vi "远端校准.vi"   [LabVIEW 2016, in "MB SLAVE.lvlib"]
uses:
  MB SLAVE.lvlib
  <vilib>/Plasmionique/MB Master/MB_Master/MB_Master.lvclass
  <vilib>/Plasmionique/MB Master/MB Master.lvlib
types:
  T1 = typedef "MB SLAVE.lvlib/启动命令类型.ctl" = enum16{"启动整机", "停止整机", "标样核查", "加标回收", "平行样测试", "零点核查", "跨度核查", "校零", "校标", "启动系统全面清洗", "水样测试", "启动采水泵阀", "校准", "仪器重启"}
  T2 = cluster{"启动类型":T1, "启动参数":enum16{"未选择", "CODMn", "氨氮", "总磷", "总氮", "CODCr"}}
  T3 = enum16{"未选择", "CODMn", "氨氮", "总磷", "总氮", "CODCr"}
  T4 = typedef "CODMn交互.ctl" = cluster{"COD浓度（mg/L)":dbl, "水样启动时间":timestamp, "加标回收启动时间":timestamp, "CODMn工作状态":enum16{"空闲", "水样测试", "标样核查", "零点核查", "跨度核查", "空白测试", "平行样测试", "加标回收", "空白校准", "标样校准", "初始化（清洗）"}, "多列列表框":i32, "平台试剂余量百分比":sgl, "关键参数":cluster{"测量量程":dbl, "测量精度":dbl, "测量间隔":dbl, "消解温度":dbl, "消解时长":dbl, "空白校准时间":timestamp, "曲线截距":dbl, "曲线斜率":dbl, "测量检出限":dbl, "测量信号值":dbl, "线性相关系数":dbl, "二次多项式系数":dbl, "标样校准时间":timestamp, "稀释倍数":dbl, "三项式系数":dbl, "空白标定系数":dbl, "量程系数":dbl, "F0/ORPA":dbl, "F1/ORPB":dbl, "F2/ORPK":dbl, "F3":dbl, "F4":dbl, "F5":dbl, "F6":dbl, "F7":dbl, "X0/滴定数":dbl, "量程":dbl}, "关键参数改变":bool, "校准信息":cluster{"低标液1浓度":dbl, "低标液1信号值":dbl, "低标液1启用":u16, "低标液2浓度":dbl, "低标液2信号值":dbl, "低标液2启用":u16, "低标液3浓度":dbl, "低标液3信号值":dbl, "低标液3启用":u16, "低标液4浓度":dbl, "低标液4信号值":dbl, "低标液4启用":u16, "低标液5浓度":dbl, "低标液5信号值":dbl, "低标液5启用":u16, "高标液1浓度":dbl, "高标液1信号值":dbl, "高标液1启用":u16, "高标液2浓度":dbl, "高标液2信号值":dbl, "高标液2启用":u16, "高标液3浓度":dbl, "高标液3信号值":dbl, "高标液3启用":u16, "高标液4浓度":dbl, "高标液4信号值":dbl, "高标液4启用":u16, "高标液5浓度":dbl, "高标液5信号值":dbl, "高标液5启用":u16, "低斜率":dbl, "低截距":dbl, "低二次多项式系数":dbl, "低线性相关系数":dbl, "高斜率":dbl, "高截距":dbl, "高二次多项式系数":dbl, "高线性相关系数":dbl}, "校准信息改变":bool, "固件版本号":string, "CODMn模块版本":T5, "协议":u16, "状态告警区":cluster{"系统时间":timestamp, "工作状态":u16, "测量模式":enum16{"待机", "连续模式", "周期模式", "定点模式", "受控模式", "手动模式"}, "告警代码":u16, "故障代码":u16, "日志代码":u16, "软件版本":u16, "F0":sgl, "F1":sgl, "F2":sgl, "F3":sgl, "T":sgl, "H":sgl, "id":u16, "flowid":u16, "量程":u16, "总磷控温温度1":sgl, "营养盐控温温度2":sgl, "ADC":sgl}, "标样核查标液浓度":dbl, "测量数据区":cluster{"空白数据时间":timestamp, "空白实测值":sgl, "标样数据时间":timestamp, "标样实测值":sgl}}
  T5 = typedef "CODMn模块版本.ctl" = enum16{"PLC版", "单片机版", "通用流路版本"}
  T6 = cluster{"系统时间":timestamp, "工作状态":u16, "测量模式":enum16{"待机", "连续模式", "周期模式", "定点模式", "受控模式", "手动模式"}, "告警代码":u16, "故障代码":u16, "日志代码":u16, "软件版本":u16, "F0":sgl, "F1":sgl, "F2":sgl, "F3":sgl, "T":sgl, "H":sgl, "id":u16, "flowid":u16, "量程":u16, "总磷控温温度1":sgl, "营养盐控温温度2":sgl, "ADC":sgl}
  T7 = typedef "氨氮交互.ctl" = cluster{"状态告警区":cluster{"系统时间":timestamp, "工作状态":u16, "测量模式":enum16{"待机", "连续模式", "周期模式", "定点模式", "受控模式", "手动模式"}, "告警代码":u16, "故障代码":u16, "日志代码":u16, "软件版本":u16, "F0":sgl, "F1":sgl, "F2":sgl, "F3":sgl, "T":sgl, "H":sgl, "id":u16, "flowid":u16, "量程":u16, "总磷控温温度1":sgl, "营养盐控温温度2":sgl, "ADC":sgl}, "平台试剂余量百分比":sgl, "关键参数":cluster{"测量量程":dbl, "测量精度":dbl, "测量间隔":dbl, "消解温度":dbl, "消解时长":dbl, "空白校准时间":timestamp, "曲线截距":dbl, "曲线斜率":dbl, "测量检出限":dbl, "测量信号值":dbl, "线性相关系数":dbl, "二次多项式系数":dbl, "标样校准时间":timestamp, "稀释倍数":dbl, "三项式系数":dbl, "空白标定系数":dbl, "量程系数":dbl, "F0/ORPA":dbl, "F1/ORPB":dbl, "F2/ORPK":dbl, "F3":dbl, "F4":dbl, "F5":dbl, "F6":dbl, "F7":dbl, "X0/滴定数":dbl, "量程":dbl}, "关键参数改变":bool, "校准信息":cluster{"低标液1浓度":dbl, "低标液1信号值":dbl, "低标液1启用":u16, "低标液2浓度":dbl, "低标液2信号值":dbl, "低标液2启用":u16, "低标液3浓度":dbl, "低标液3信号值":dbl, "低标液3启用":u16, "低标液4浓度":dbl, "低标液4信号值":dbl, "低标液4启用":u16, "低标液5浓度":dbl, "低标液5信号值":dbl, "低标液5启用":u16, "高标液1浓度":dbl, "高标液1信号值":dbl, "高标液1启用":u16, "高标液2浓度":dbl, "高标液2信号值":dbl, "高标液2启用":u16, "高标液3浓度":dbl, "高标液3信号值":dbl, "高标液3启用":u16, "高标液4浓度":dbl, "高标液4信号值":dbl, "高标液4启用":u16, "高标液5浓度":dbl, "高标液5信号值":dbl, "高标液5启用":u16, "低斜率":dbl, "低截距":dbl, "低二次多项式系数":dbl, "低线性相关系数":dbl, "高斜率":dbl, "高截距":dbl, "高二次多项式系数":dbl, "高线性相关系数":dbl}, "校准信息改变":bool, "固件版本号":string}
  T8 = typedef "总磷交互.ctl" = cluster{"状态告警区":cluster{"系统时间":timestamp, "工作状态":u16, "测量模式":enum16{"待机", "连续模式", "周期模式", "定点模式", "受控模式", "手动模式"}, "告警代码":u16, "故障代码":u16, "日志代码":u16, "软件版本":u16, "F0":sgl, "F1":sgl, "F2":sgl, "F3":sgl, "T":sgl, "H":sgl, "id":u16, "flowid":u16, "量程":u16, "总磷控温温度1":sgl, "营养盐控温温度2":sgl, "ADC":sgl}, "平台试剂余量百分比":sgl, "关键参数":cluster{"测量量程":dbl, "测量精度":dbl, "测量间隔":dbl, "消解温度":dbl, "消解时长":dbl, "空白校准时间":timestamp, "曲线截距":dbl, "曲线斜率":dbl, "测量检出限":dbl, "测量信号值":dbl, "线性相关系数":dbl, "二次多项式系数":dbl, "标样校准时间":timestamp, "稀释倍数":dbl, "三项式系数":dbl, "空白标定系数":dbl, "量程系数":dbl, "F0/ORPA":dbl, "F1/ORPB":dbl, "F2/ORPK":dbl, "F3":dbl, "F4":dbl, "F5":dbl, "F6":dbl, "F7":dbl, "X0/滴定数":dbl, "量程":dbl}, "关键参数改变":bool, "校准信息":cluster{"低标液1浓度":dbl, "低标液1信号值":dbl, "低标液1启用":u16, "低标液2浓度":dbl, "低标液2信号值":dbl, "低标液2启用":u16, "低标液3浓度":dbl, "低标液3信号值":dbl, "低标液3启用":u16, "低标液4浓度":dbl, "低标液4信号值":dbl, "低标液4启用":u16, "低标液5浓度":dbl, "低标液5信号值":dbl, "低标液5启用":u16, "高标液1浓度":dbl, "高标液1信号值":dbl, "高标液1启用":u16, "高标液2浓度":dbl, "高标液2信号值":dbl, "高标液2启用":u16, "高标液3浓度":dbl, "高标液3信号值":dbl, "高标液3启用":u16, "高标液4浓度":dbl, "高标液4信号值":dbl, "高标液4启用":u16, "高标液5浓度":dbl, "高标液5信号值":dbl, "高标液5启用":u16, "低斜率":dbl, "低截距":dbl, "低二次多项式系数":dbl, "低线性相关系数":dbl, "高斜率":dbl, "高截距":dbl, "高二次多项式系数":dbl, "高线性相关系数":dbl}, "校准信息改变":bool, "固件版本号":string}
  T9 = typedef "总氮交互.ctl" = cluster{"状态告警区":cluster{"系统时间":timestamp, "工作状态":u16, "测量模式":enum16{"待机", "连续模式", "周期模式", "定点模式", "受控模式", "手动模式"}, "告警代码":u16, "故障代码":u16, "日志代码":u16, "软件版本":u16, "F0":sgl, "F1":sgl, "F2":sgl, "F3":sgl, "T":sgl, "H":sgl, "id":u16, "flowid":u16, "量程":u16, "总磷控温温度1":sgl, "营养盐控温温度2":sgl, "ADC":sgl}, "平台试剂余量百分比":sgl, "关键参数":cluster{"测量量程":dbl, "测量精度":dbl, "测量间隔":dbl, "消解温度":dbl, "消解时长":dbl, "空白校准时间":timestamp, "曲线截距":dbl, "曲线斜率":dbl, "测量检出限":dbl, "测量信号值":dbl, "线性相关系数":dbl, "二次多项式系数":dbl, "标样校准时间":timestamp, "稀释倍数":dbl, "三项式系数":dbl, "空白标定系数":dbl, "量程系数":dbl, "F0/ORPA":dbl, "F1/ORPB":dbl, "F2/ORPK":dbl, "F3":dbl, "F4":dbl, "F5":dbl, "F6":dbl, "F7":dbl, "X0/滴定数":dbl, "量程":dbl}, "关键参数改变":bool, "校准信息":cluster{"低标液1浓度":dbl, "低标液1信号值":dbl, "低标液1启用":u16, "低标液2浓度":dbl, "低标液2信号值":dbl, "低标液2启用":u16, "低标液3浓度":dbl, "低标液3信号值":dbl, "低标液3启用":u16, "低标液4浓度":dbl, "低标液4信号值":dbl, "低标液4启用":u16, "低标液5浓度":dbl, "低标液5信号值":dbl, "低标液5启用":u16, "高标液1浓度":dbl, "高标液1信号值":dbl, "高标液1启用":u16, "高标液2浓度":dbl, "高标液2信号值":dbl, "高标液2启用":u16, "高标液3浓度":dbl, "高标液3信号值":dbl, "高标液3启用":u16, "高标液4浓度":dbl, "高标液4信号值":dbl, "高标液4启用":u16, "高标液5浓度":dbl, "高标液5信号值":dbl, "高标液5启用":u16, "低斜率":dbl, "低截距":dbl, "低二次多项式系数":dbl, "低线性相关系数":dbl, "高斜率":dbl, "高截距":dbl, "高二次多项式系数":dbl, "高线性相关系数":dbl}, "校准信息改变":bool, "固件版本号":string}
  T10 = typedef "CODCr交互.ctl" = cluster{"状态告警区":cluster{"系统时间":timestamp, "工作状态":u16, "测量模式":enum16{"待机", "连续模式", "周期模式", "定点模式", "受控模式", "手动模式"}, "告警代码":u16, "故障代码":u16, "日志代码":u16, "软件版本":u16, "F0":sgl, "F1":sgl, "F2":sgl, "F3":sgl, "T":sgl, "H":sgl, "id":u16, "flowid":u16, "量程":u16, "总磷控温温度1":sgl, "营养盐控温温度2":sgl, "ADC":sgl}, "平台试剂余量百分比":sgl, "关键参数":cluster{"测量量程":dbl, "测量精度":dbl, "测量间隔":dbl, "消解温度":dbl, "消解时长":dbl, "空白校准时间":timestamp, "曲线截距":dbl, "曲线斜率":dbl, "测量检出限":dbl, "测量信号值":dbl, "线性相关系数":dbl, "二次多项式系数":dbl, "标样校准时间":timestamp, "稀释倍数":dbl, "三项式系数":dbl, "空白标定系数":dbl, "量程系数":dbl, "F0/ORPA":dbl, "F1/ORPB":dbl, "F2/ORPK":dbl, "F3":dbl, "F4":dbl, "F5":dbl, "F6":dbl, "F7":dbl, "X0/滴定数":dbl, "量程":dbl}, "关键参数改变":bool, "校准信息":cluster{"低标液1浓度":dbl, "低标液1信号值":dbl, "低标液1启用":u16, "低标液2浓度":dbl, "低标液2信号值":dbl, "低标液2启用":u16, "低标液3浓度":dbl, "低标液3信号值":dbl, "低标液3启用":u16, "低标液4浓度":dbl, "低标液4信号值":dbl, "低标液4启用":u16, "低标液5浓度":dbl, "低标液5信号值":dbl, "低标液5启用":u16, "高标液1浓度":dbl, "高标液1信号值":dbl, "高标液1启用":u16, "高标液2浓度":dbl, "高标液2信号值":dbl, "高标液2启用":u16, "高标液3浓度":dbl, "高标液3信号值":dbl, "高标液3启用":u16, "高标液4浓度":dbl, "高标液4信号值":dbl, "高标液4启用":u16, "高标液5浓度":dbl, "高标液5信号值":dbl, "高标液5启用":u16, "低斜率":dbl, "低截距":dbl, "低二次多项式系数":dbl, "低线性相关系数":dbl, "高斜率":dbl, "高截距":dbl, "高二次多项式系数":dbl, "高线性相关系数":dbl}, "校准信息改变":bool, "固件版本号":string}
  T11 = cluster{"空白数据时间":timestamp, "空白实测值":sgl, "标样数据时间":timestamp, "标样实测值":sgl}
  T12 = typedef "SingleStepTestV3.lvlib/SingleStepTestV3.lvclass/仪器版本.ctl" = enum16{"V3.1版", "V4版", "V3版", "V4.2版"}
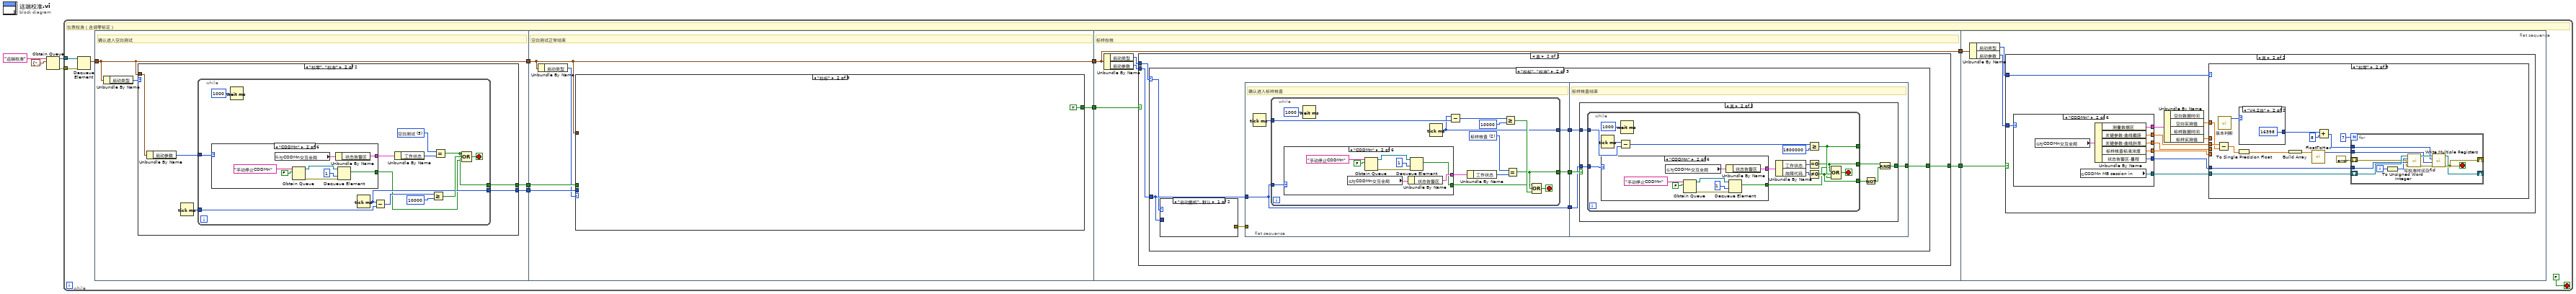
[diagram p0: block diagram]
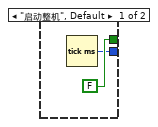
[diagram p2: hidden frame]
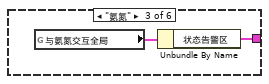
[diagram p4: hidden frame]
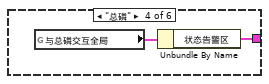
[diagram p5: hidden frame]
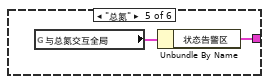
[diagram p6: hidden frame]
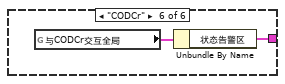
[diagram p7: hidden frame]
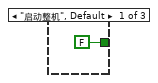
[diagram p8: hidden frame]
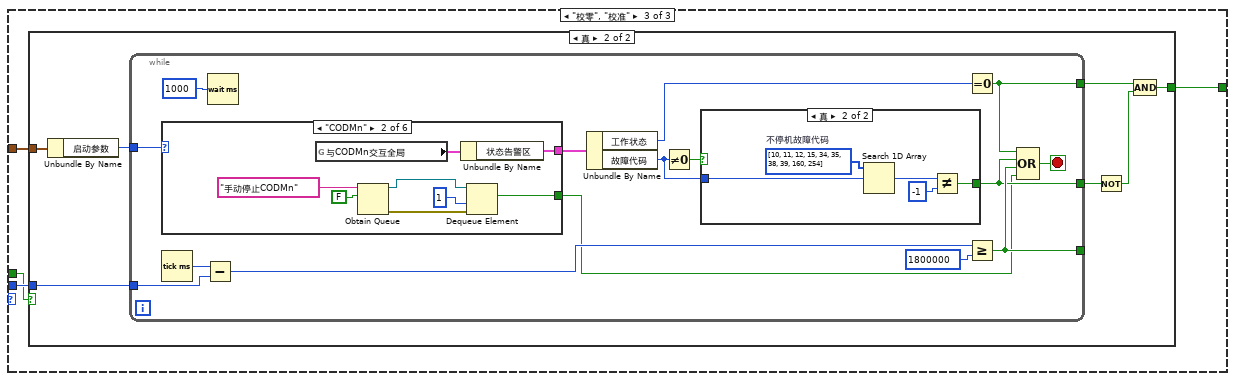
[diagram p9: hidden frame]
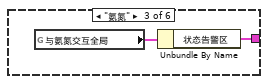
[diagram p13: hidden frame]
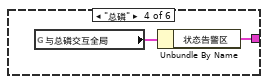
[diagram p14: hidden frame]
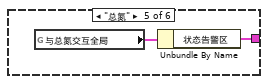
[diagram p15: hidden frame]
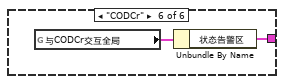
[diagram p16: hidden frame]
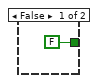
[diagram p17: hidden frame]
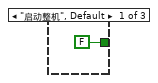
[diagram p18: hidden frame]
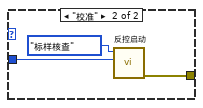
[diagram p19: hidden frame]
diagram:
  n1 = Obtain Queue(name (unnamed)="远端校准" ("名称（未命名）"), element data type=T2 {"启动类型"=enum."校零", "启动参数"=enum."CODMn"}) -> (queue out=w3:refnum<queue>, error out=w2:errorcluster)  [unwired: 3 in, 1 out]
  n2 = while {
    tunnel: w3 -> [w15]
    tunnel: w2 -> [w14]
    stop <- FALSE stop-if-true
    # "仪表校准（含调零标定）"
    n3 = Dequeue Element(queue=w15, error in (no error)=w14) -> (element=w12:T2)  [unwired: 1 in, 3 out]
    n4 = flat-sequence {
      tunnel: w12 -> [w17]
      tunnel: [w17] -> w11
      tunnel: [w19] -> w10
      tunnel: [w18] -> w9
      tunnel: w11 -> [w57]
      tunnel: w10 -> [w60]
      tunnel: w9 -> [w59]
      tunnel: [w57] -> w6
      tunnel: [w56] -> w5
      tunnel: [w114] -> w8
      tunnel: [w113] -> w7
      tunnel: w6 -> [w113]
      tunnel: w5 -> [w112]
      tunnel: w8 -> [w206]
      tunnel: w7 -> [w207]
      frame #0 {
        # "确认进入空白测试"
        n5 = Unbundle By Name(w17) -> ("启动类型"=w16:T1)
        n6 = case shown="\"校零\", \"校准\"" w16 {
          tunnel: [w20 w25] -> w19
          tunnel: [FALSE w24] -> w18
          tunnel: w17 -> [_ w22]
          frame "启动整机", Default {
            n7 = Tick Count (ms)() -> (millisecond timer value=w20:u32)
          }
          frame "校零", "校准" {
            n8 = Unbundle By Name(w22) -> ("启动参数"=w23:T3)
            n9 = Tick Count (ms)() -> (millisecond timer value=w26:u32)
            n10 = while {
              tunnel: w23 -> [w39]
              tunnel: w26 -> [w37]
              tunnel: [w29] -> w25
              tunnel: [w28] -> w24
              stop <- w33 stop-if-true
              w31 = u16 5 items=["空闲"=0, "水样测试"=1, "标样核查"=2, "零点核查"=3, "跨度核查"=4, "空白测试"=5, "平行样测试"=6, "加标回收"=7, "空白校准"=8, "标样校准"=9, "初始化（清洗）"=10, "单步调试"=254, "简易流程"=255] ("工作状态")
              n11 = case shown="\"CODMn\"" w39 {
                tunnel: [_ w46 w48 w50 w52 w54] -> w38
                tunnel: [_ w40 _ _ _ _] -> w27
                frame "未选择", Default {
                }
                frame "CODMn" {
                  n12 = global read "modbus slave全局.vi" "与CODMn交互全局"() -> (w47:T4)
                  n13 = Obtain Queue(name (unnamed)="手动停止CODMn" ("名称（未命名）"), element data type=FALSE) -> (queue out=w43:refnum<queue>, error out=w44:errorcluster)  [unwired: 3 in, 1 out]
                  n14 = Unbundle By Name(w47) -> ("状态告警区"=w46:T6)
                  n15 = Dequeue Element(queue=w43, timeout in ms (-1)=1 ("超时毫秒(-1)"), error in (no error)=w44) -> (element=w40:bool)  [unwired: 3 out]
                }
                frame "氨氮" {
                  n16 = global read "modbus slave全局.vi" "与氨氮交互全局"() -> (w49:T7)
                  n17 = Unbundle By Name(w49) -> ("状态告警区"=w48:T6)
                }
                frame "总磷" {
                  n18 = global read "modbus slave全局.vi" "与总磷交互全局"() -> (w51:T8)
                  n19 = Unbundle By Name(w51) -> ("状态告警区"=w50:T6)
                }
                frame "总氮" {
                  n20 = global read "modbus slave全局.vi" "与总氮交互全局"() -> (w53:T9)
                  n21 = Unbundle By Name(w53) -> ("状态告警区"=w52:T6)
                }
                frame "CODCr" {
                  n22 = global read "modbus slave全局.vi" "与CODCr交互全局"() -> (w55:T10)
                  n23 = Unbundle By Name(w55) -> ("状态告警区"=w54:T6)
                }
              }
              n24 = Wait (ms)(milliseconds to wait=u32 1000 ("等待时间（毫秒）")) -> ()  [unwired: 1 out]
              n25 = Tick Count (ms)() -> (millisecond timer value=w29:u32)
              n26 = Subtract(x=w29, y=w37) -> (x-y=w35:u32)
              n27 = Unbundle By Name(w38) -> ("工作状态"=w30:u16)
              n28 = Greater Or Equal?(x=w35, y=u32 10000) -> (x >= y?=w32:bool)
              n29 = Equal?(x=w31, y=w30) -> (x = y?=w28:bool)
              n30 = Compound Arithmetic op=OR ("复合运算")(w28, w32, w27) -> (w33:bool)
            }
          }
        }
      }
      frame #1 {
        # "空白测试正常结束"
        n31 = Unbundle By Name(w57) -> ("启动类型"=w58:T1)
        n32 = case shown="\"校标\"" w58 {
          tunnel: w60 -> [_ _ w66]
          tunnel: w59 -> [_ _ w65]
          tunnel: [FALSE TRUE w64] -> w56
          tunnel: w57 -> [_ _ w63]
          frame "启动整机", Default {
          }
          frame "校标" {
          }
          frame "校零", "校准" {
            n33 = case shown="真" w65 {
              tunnel: w66 -> [_ w73]
              tunnel: w63 -> [_ w68]
              tunnel: [_ w69] -> w64
              frame False {
              }
              frame True {
                n34 = Unbundle By Name(w68) -> ("启动参数"=w67:T3)
                n35 = while {
                  tunnel: w73 -> [w86]
                  tunnel: [w75] -> w72
                  tunnel: [w80] -> _
                  tunnel: [w79] -> w70
                  tunnel: w67 -> [w78]
                  stop <- w81 stop-if-true
                  n36 = case shown="\"CODMn\"" w78 {
                    tunnel: [_ w100 w102 w104 w106 w108] -> w88
                    tunnel: [_ w94 _ _ _ _] -> w74
                    frame "未选择", Default {
                    }
                    frame "CODMn" {
                      n37 = global read "modbus slave全局.vi" "与CODMn交互全局"() -> (w101:T4)
                      n38 = Obtain Queue(name (unnamed)="手动停止CODMn" ("名称（未命名）"), element data type=FALSE) -> (queue out=w97:refnum<queue>, error out=w98:errorcluster)  [unwired: 3 in, 1 out]
                      n39 = Unbundle By Name(w101) -> ("状态告警区"=w100:T6)
                      n40 = Dequeue Element(queue=w97, timeout in ms (-1)=1 ("超时毫秒(-1)"), error in (no error)=w98) -> (element=w94:bool)  [unwired: 3 out]
                    }
                    frame "氨氮" {
                      n41 = global read "modbus slave全局.vi" "与氨氮交互全局"() -> (w103:T7)
                      n42 = Unbundle By Name(w103) -> ("状态告警区"=w102:T6)
                    }
                    frame "总磷" {
                      n43 = global read "modbus slave全局.vi" "与总磷交互全局"() -> (w105:T8)
                      n44 = Unbundle By Name(w105) -> ("状态告警区"=w104:T6)
                    }
                    frame "总氮" {
                      n45 = global read "modbus slave全局.vi" "与总氮交互全局"() -> (w107:T9)
                      n46 = Unbundle By Name(w107) -> ("状态告警区"=w106:T6)
                    }
                    frame "CODCr" {
                      n47 = global read "modbus slave全局.vi" "与CODCr交互全局"() -> (w109:T10)
                      n48 = Unbundle By Name(w109) -> ("状态告警区"=w108:T6)
                    }
                  }
                  n49 = Tick Count (ms)() -> (millisecond timer value=w87:u32)
                  n50 = Subtract(x=w87, y=w86) -> (x-y=w84:u32)
                  n51 = Wait (ms)(milliseconds to wait=u32 1000 ("等待时间（毫秒）")) -> ()  [unwired: 1 out]
                  n52 = Unbundle By Name(w88) -> ("工作状态"=w82:u16, "故障代码"=w76:u16)
                  n53 = Not Equal To 0?(x=w76) -> (x != 0?=w77:bool)
                  n54 = case shown="真" w77 {
                    tunnel: w76 -> [_ w92]
                    tunnel: [_ w89] -> w75
                    frame False {
                    }
                    frame True {
                      w93 = u16[] [10, 11, 12, 15, 34, 35, 38, 39, 160, 254]  # 不停机故障代码
                      n55 = Search 1D Array(1D array=w93, element=w92) -> (index of element=w91:i32)  [unwired: 1 in]
                      n56 = Not Equal?(x=w91, y=-1) -> (x != y?=w89:bool)
                    }
                  }
                  n57 = Equal To 0?(x=w82) -> (x = 0?=w79:bool)
                  n58 = Greater Or Equal?(x=w84, y=u32 1800000) -> (x >= y?=w80:bool)
                  n59 = Compound Arithmetic op=OR ("复合运算")(w79, w75, w80, w74) -> (w81:bool)
                }
                n60 = Not(x=w72) -> (.not. x?=w71:bool)
                n61 = Compound Arithmetic op=AND ("复合运算")(w70, w71) -> (w69:bool)
              }
            }
          }
        }
      }
      frame #2 {
        # "标样校核"
        n62 = Unbundle By Name(w113) -> ("启动类型"=w111:T1, "启动参数"=w110:T3)
        n63 = case shown="真" w112 {
          tunnel: w111 -> [_ w118]
          tunnel: w110 -> [_ w117]
          tunnel: [FALSE w116] -> w114
          frame False {
          }
          frame True {
            n64 = case shown="\"校标\", \"校准\"" w118 {
              selector: w118 -> [_ w120 _]
              tunnel: w117 -> [_ w125 _]
              tunnel: [FALSE w121 TRUE] -> w116
              frame "启动整机", Default {
              }
              frame "校标", "校准" {
                n65 = case shown="\"启动整机\", 默认" w120 {
                  tunnel: [_ w128] -> w126
                  tunnel: w125 -> [_ w127]
                  frame "启动整机", Default {
                  }
                  frame "校准" {
                    n66 = call "反控启动.vi"("启动参数"=w127, "启动类型"=启动命令类型."标样核查") -> ("error out"=w128:errorcluster)  [unwired: 9 in]
                  }
                }
                n67 = flat-sequence {
                  tunnel: w126 -> [_]
                  tunnel: w125 -> [w130]
                  tunnel: [w132] -> w124
                  tunnel: [w131] -> w123
                  tunnel: [w130] -> w122
                  tunnel: w124 -> [w166]
                  tunnel: w123 -> [w165]
                  tunnel: w122 -> [w164]
                  tunnel: [w163] -> w121
                  frame #0 {
                    # "确认进入标样核查"
                    n68 = Tick Count (ms)() -> (millisecond timer value=w133:u32)
                    n69 = while {
                      tunnel: w130 -> [w146]
                      tunnel: w133 -> [w144]
                      tunnel: [w136] -> w131
                      tunnel: [w135] -> w132
                      stop <- w140 stop-if-true
                      w138 = u16 2 items=["空闲"=0, "水样测试"=1, "标样核查"=2, "零点核查"=3, "跨度核查"=4, "空白测试"=5, "平行样测试"=6, "加标回收"=7, "空白校准"=8, "标样校准"=9, "初始化（清洗）"=10, "单步调试"=254, "简易流程"=255] ("工作状态")
                      n70 = case shown="\"CODMn\"" w146 {
                        tunnel: [_ w153 w155 w157 w159 w161] -> w145
                        tunnel: [_ w147 _ _ _ _] -> w134
                        frame "未选择", Default {
                        }
                        frame "CODMn" {
                          n71 = global read "modbus slave全局.vi" "与CODMn交互全局"() -> (w154:T4)
                          n72 = Obtain Queue(name (unnamed)="手动停止CODMn" ("名称（未命名）"), element data type=FALSE) -> (queue out=w150:refnum<queue>, error out=w149:errorcluster)  [unwired: 3 in, 1 out]
                          n73 = Unbundle By Name(w154) -> ("状态告警区"=w153:T6)
                          n74 = Dequeue Element(queue=w150, timeout in ms (-1)=1 ("超时毫秒(-1)"), error in (no error)=w149) -> (element=w147:bool)  [unwired: 3 out]
                        }
                        frame "氨氮" {
                          n75 = global read "modbus slave全局.vi" "与氨氮交互全局"() -> (w156:T7)
                          n76 = Unbundle By Name(w156) -> ("状态告警区"=w155:T6)
                        }
                        frame "总磷" {
                          n77 = global read "modbus slave全局.vi" "与总磷交互全局"() -> (w158:T8)
                          n78 = Unbundle By Name(w158) -> ("状态告警区"=w157:T6)
                        }
                        frame "总氮" {
                          n79 = global read "modbus slave全局.vi" "与总氮交互全局"() -> (w160:T9)
                          n80 = Unbundle By Name(w160) -> ("状态告警区"=w159:T6)
                        }
                        frame "CODCr" {
                          n81 = global read "modbus slave全局.vi" "与CODCr交互全局"() -> (w162:T10)
                          n82 = Unbundle By Name(w162) -> ("状态告警区"=w161:T6)
                        }
                      }
                      n83 = Wait (ms)(milliseconds to wait=u32 1000 ("等待时间（毫秒）")) -> ()  [unwired: 1 out]
                      n84 = Tick Count (ms)() -> (millisecond timer value=w136:u32)
                      n85 = Subtract(x=w136, y=w144) -> (x-y=w142:u32)
                      n86 = Unbundle By Name(w145) -> ("工作状态"=w137:u16)
                      n87 = Greater Or Equal?(x=w142, y=u32 10000) -> (x >= y?=w139:bool)
                      n88 = Equal?(x=w138, y=w137) -> (x = y?=w135:bool)
                      n89 = Compound Arithmetic op=OR ("复合运算")(w134, w135, w139) -> (w140:bool)
                    }
                  }
                  frame #1 {
                    # "标样核查结束"
                    n90 = case shown="真" w166 {
                      tunnel: w165 -> [_ w172]
                      tunnel: [_ w168] -> w163
                      tunnel: w164 -> [_ w167]
                      frame False {
                      }
                      frame True {
                        n91 = while {
                          tunnel: w172 -> [w183]
                          tunnel: [w177] -> w171
                          tunnel: [w176] -> _
                          tunnel: [w175] -> w169
                          tunnel: w167 -> [w174]
                          stop <- w178 stop-if-true
                          n92 = Tick Count (ms)() -> (millisecond timer value=w184:u32)
                          n93 = case shown="\"CODMn\"" w174 {
                            tunnel: [_ w193 w195 w197 w199 w201] -> w186
                            tunnel: [_ w187 _ _ _ _] -> w173
                            frame "未选择", Default {
                            }
                            frame "CODMn" {
                              n94 = global read "modbus slave全局.vi" "与CODMn交互全局"() -> (w194:T4)
                              n95 = Obtain Queue(name (unnamed)="手动停止CODMn" ("名称（未命名）"), element data type=FALSE) -> (queue out=w190:refnum<queue>, error out=w189:errorcluster)  [unwired: 3 in, 1 out]
                              n96 = Unbundle By Name(w194) -> ("状态告警区"=w193:T6)
                              n97 = Dequeue Element(queue=w190, timeout in ms (-1)=1 ("超时毫秒(-1)"), error in (no error)=w189) -> (element=w187:bool)  [unwired: 3 out]
                            }
                            frame "氨氮" {
                              n98 = global read "modbus slave全局.vi" "与氨氮交互全局"() -> (w196:T7)
                              n99 = Unbundle By Name(w196) -> ("状态告警区"=w195:T6)
                            }
                            frame "总磷" {
                              n100 = global read "modbus slave全局.vi" "与总磷交互全局"() -> (w198:T8)
                              n101 = Unbundle By Name(w198) -> ("状态告警区"=w197:T6)
                            }
                            frame "总氮" {
                              n102 = global read "modbus slave全局.vi" "与总氮交互全局"() -> (w200:T9)
                              n103 = Unbundle By Name(w200) -> ("状态告警区"=w199:T6)
                            }
                            frame "CODCr" {
                              n104 = global read "modbus slave全局.vi" "与CODCr交互全局"() -> (w202:T10)
                              n105 = Unbundle By Name(w202) -> ("状态告警区"=w201:T6)
                            }
                          }
                          n106 = Subtract(x=w184, y=w183) -> (x-y=w181:u32)
                          n107 = Wait (ms)(milliseconds to wait=u32 1000 ("等待时间（毫秒）")) -> ()  [unwired: 1 out]
                          n108 = Unbundle By Name(w186) -> ("工作状态"=w179:u16, "故障代码"=w185:u16)
                          n109 = Greater Or Equal?(x=w181, y=u32 1800000) -> (x >= y?=w176:bool)
                          n110 = Equal To 0?(x=w179) -> (x = 0?=w175:bool)
                          n111 = Not Equal To 0?(x=w185) -> (x != 0?=w177:bool)
                          n112 = Compound Arithmetic op=OR ("复合运算")(w173, w175, w177, w176) -> (w178:bool)
                        }
                        n113 = Not(x=w171) -> (.not. x?=w170:bool)
                        n114 = Compound Arithmetic op=AND ("复合运算")(w169, w170) -> (w168:bool)
                      }
                    }
                  }
                }
              }
              frame "校零" {
              }
            }
          }
        }
      }
      frame #3 {
        n115 = Unbundle By Name(w207) -> ("启动类型"=w204:T1, "启动参数"=w205:T3)
        n116 = case shown="真" w206 {
          tunnel: w205 -> [_ w217]
          tunnel: w204 -> [_ w215]
          frame False {
          }
          frame True {
            n117 = case shown="\"CODMn\"" w217 {
              tunnel: [_ w290 _ _ _ _] -> w216
              tunnel: [_ w289 _ _ _ _] -> w213
              tunnel: [_ w288 _ _ _ _] -> w212
              tunnel: [_ w287 _ _ _ _] -> w210
              tunnel: [_ w286 _ _ _ _] -> w209
              tunnel: [_ w285 _ _ _ _] -> w208
              frame "未选择", Default {
              }
              frame "CODMn" {
                n118 = global read "modbus slave全局.vi" "与CODMn交互全局"() -> (w291:T4)
                n119 = global read "modbus slave全局.vi" "CODMn MB session in"() -> (w287:refnum<class "MB_Master.lvclass">)
                n120 = Unbundle By Name(w291) -> ("测量数据区"=w290:T11, "关键参数.曲线截距"=w289:dbl, "关键参数.曲线斜率"=w288:dbl, "标样核查标液浓度"=w286:dbl, "状态告警区.量程"=w285:u16)
              }
              frame "氨氮" {
              }
              frame "总磷" {
                n121 = global read "modbus slave全局.vi" "与总磷交互全局"() -> (w292:T8)
                n122 = Unbundle By Name(w292) -> ()  [unwired: 1 out]
              }
              frame "总氮" {
                n123 = global read "modbus slave全局.vi" "与总氮交互全局"() -> (w293:T9)
                n124 = Unbundle By Name(w293) -> ()  [unwired: 1 out]
              }
              frame "CODCr" {
                n125 = global read "modbus slave全局.vi" "与CODCr交互全局"() -> (w294:T10)
                n126 = Unbundle By Name(w294) -> ()  [unwired: 1 out]
              }
            }
            n127 = Unbundle By Name(w216) -> ("空白实测值"=w214:sgl, "标样实测值"=w211:sgl)  [unwired: 2 out]
            n128 = case shown="\"校零\"" w215 {
              tunnel: w214 -> [_ w230 _]
              tunnel: w213 -> [_ w231 w266]
              tunnel: w212 -> [_ _ w264]
              tunnel: w211 -> [_ _ w268]
              tunnel: w210 -> [_ w221 w259]
              tunnel: w209 -> [_ _ w267]
              tunnel: w208 -> [_ w220 w258]
              frame "启动整机", Default {
              }
              frame "校零" {
                n129 = Subtract(x=w231, y=w230) -> (x-y=w228:dbl)
                n130 = call "版本判断.vi"() -> ("仪器版本"=w229:T12)  [unwired: 11 in]
                n131 = To Single Precision Float(number=w228) -> (single precision float=w227:sgl)
                n132 = case shown="\"V4.2版\"" w229 {
                  tunnel: [u16 8234 ("starting address") u16 16398 ("starting address")] -> w225
                  frame "V3.1版", Default {
                  }
                  frame "V4.2版" {
                  }
                }
                n133 = Build Array(w227) -> (w226:sgl[])
                n134 = call "FloatToHex.vi"("浮点数"=w226) -> ("DCBA整形输出"=w218:u16[])  [unwired: 10 in]
                n135 = Add(x=w225, y=u16 8) -> (x+y=w219:u16)
                n136 = for {
                  N: 7 -> [_]
                  tunnel: w220 -> [w241]
                  shift-right: [w233] -> _
                  shift-left: errorcluster {"status"=FALSE, "code"=0, "source"=""} ("error in (no error)") -> [w240]
                  tunnel: w219 -> [w235]
                  tunnel: w218 -> [w234]
                  shift-right: [w232] -> _
                  shift-left: w221 -> [w242]
                  i -> [w238]
                  stop <- w233 stop-if-true
                  n137 = To Unsigned Word Integer(number=w238) -> (unsigned 16bit integer=w237:u16)
                  n138 = call "写校准时间及fid.vi"("error in (no error)"=w240, "量程"=w241, "fid"=w237, "MB session in"=w242) -> ("error out"=w236:errorcluster, "MB session out"=w239:refnum<class "MB_Master.lvclass">)  [unwired: 6 in]
                  n139 = call <vilib>:"Write Multiple Registers.vi"("error in (no error)"=w236, "values"=w234, "starting address"=w235, "MB session in"=w239) -> ("error out"=w233:errorcluster, "MB session out"=w232:refnum<class "MB_Master.lvclass">)  [unwired: 6 in]
                }
              }
              frame "校标", "校准" {
                n140 = Divide(x=w268, y=w267) -> (x/y=w265:dbl)
                n141 = Multiply(x=w264, y=w265) -> (x*y=w254:dbl)
                n142 = Multiply(x=w265, y=w266) -> (x*y=w247:dbl)
                n143 = call "版本判断.vi"() -> ("仪器版本"=w272:T12)  [unwired: 11 in]
                n144 = Number To Fractional String(number=w254, precision (6)=i16 6 ("精度(6)")) -> (F-format string=w251:string)  [unwired: 2 in]
                n145 = Number To Fractional String(number=w247, precision (6)=i16 6 ("精度(6)")) -> (F-format string=w250:string)  [unwired: 2 in]
                n146 = case shown="\"V4.2版\"" w272 {
                  tunnel: [u16 8234 ("starting address") u16 16398 ("starting address")] -> w270
                  frame "V3.1版", Default {
                  }
                  frame "V4.2版" {
                  }
                }
                n147 = Fract/Exp String To Number(string=w251, default (0 dbl)=sgl 0.0) -> (number=w246:sgl)  [unwired: 2 in, 1 out]
                n148 = Fract/Exp String To Number(string=w250, default (0 dbl)=sgl 0.0) -> (number=w245:sgl)  [unwired: 2 in, 1 out]
                n149 = Build Array(w246) -> (w271:sgl[])
                n150 = Build Array(w245) -> (w263:sgl[])
                n151 = call "FloatToHex.vi"("浮点数"=w271) -> ("DCBA整形输出"=w262:u16[])  [unwired: 10 in]
                n152 = call "FloatToHex.vi"("浮点数"=w263) -> ("DCBA整形输出"=w261:u16[])  [unwired: 10 in]
                n153 = Build Array (concatenate)(w262, w261) -> (w255:u16[])
                n154 = Add(x=w270, y=u16 4) -> (x+y=w256:u16)
                n155 = for {
                  N: 7 -> [_]
                  tunnel: w258 -> [w281]
                  shift-right: [w274] -> _
                  shift-left: errorcluster {"status"=FALSE, "code"=0, "source"=""} ("error in (no error)") -> [w280]
                  tunnel: w256 -> [w278]
                  tunnel: w255 -> [w277]
                  shift-right: [w273] -> _
                  shift-left: w259 -> [w282]
                  i -> [w276]
                  stop <- w274 stop-if-true
                  n156 = To Unsigned Word Integer(number=w276) -> (unsigned 16bit integer=w275:u16)
                  n157 = call "写校准时间及fid.vi"("error in (no error)"=w280, "量程"=w281, "fid"=w275, "MB session in"=w282) -> ("error out"=w274:errorcluster, "MB session out"=w279:refnum<class "MB_Master.lvclass">)  [unwired: 6 in]
                  n158 = call <vilib>:"Write Multiple Registers.vi"("error in (no error)"=w274, "values"=w277, "starting address"=w278, "MB session in"=w279) -> ("MB session out"=w273:refnum<class "MB_Master.lvclass">)  [unwired: 6 in, 1 out]
                }
              }
            }
          }
        }
      }
    }
  }
